vi "Write DBL Value.vi"(8 "error in (no error)":errorcluster, 10 "DBL Value":dbl, 11 "Acquired Result in":refnum<class "Acquired Result.lvclass">) -> (0 "error out":errorcluster, 3 "Acquired Result out":refnum<class "Acquired Result.lvclass">)   [LabVIEW 2016, in "Acquired Result.lvclass"]
uses:
  Acquired Result.lvclass
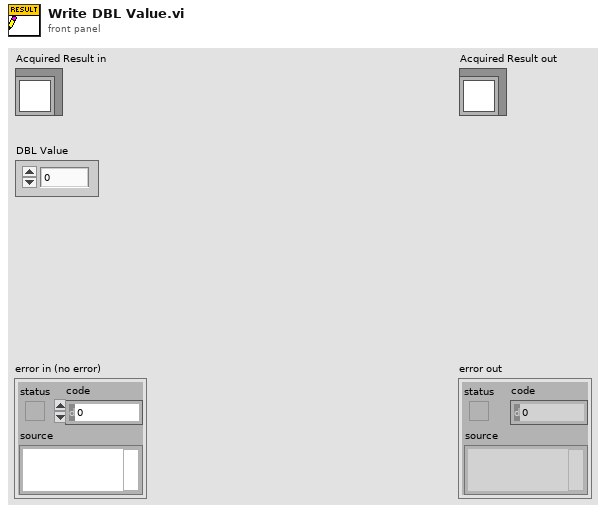
[diagram p1: front panel]
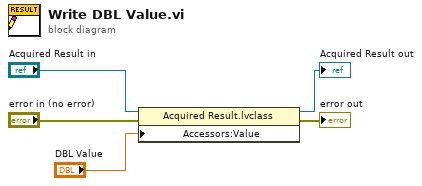
[diagram p0: block diagram]
diagram:
  n1 = property class="Acquired Result.lvclass"(reference="Acquired Result in", error in="error in (no error)", "Accessors:Value"="DBL Value") -> (reference out=→"Acquired Result out":refnum<class "Acquired Result.lvclass">, error out=→"error out":errorcluster)
